vi "SQLDisconnect.vi"(4 "error in (no error)":errorcluster, 7 "InputHandle":i32) -> (0 "error out":errorcluster, 3 "OutputHandle":i32)   [LabVIEW 2011]
doc: "Se déconnecte de la base de donnée référencée par le lien"
uses:
  Odbc32.dll
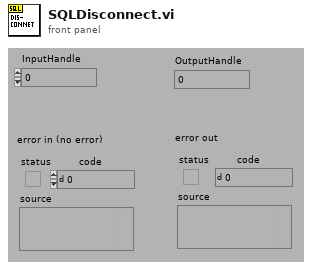
[diagram p1: front panel]
types:
  T1 = enum16{"NOPE", "SQL_HANDLE_ENV", "SQL_HANDLE_DBC", "SQL_HANDLE_STMT", "SQL_HANDLE_DESC"}
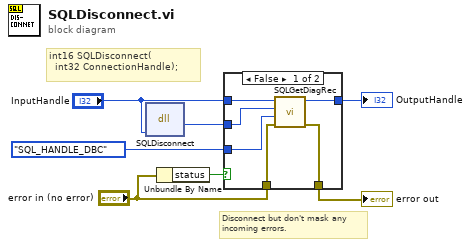
[diagram p0: block diagram]
diagram:
  # "Disconnect but don't mask any\nincoming errors."
  # "int16 SQLDisconnect(\n  int32 ConnectionHandle);"
  n1 = dll-call lib="Odbc32.dll" fn="SQLDisconnect"("ConnectionHandle"="InputHandle") -> (w4:i16)  [unwired: 4 in, 2 out]
  n2 = Unbundle By Name("error in (no error)") -> ("status"=w2:bool)
  n3 = case shown="False" w2 {
    tunnel: "error in (no error)" -> [w13 w15]
    tunnel: [w12 w15] -> w7
    tunnel: "InputHandle" -> [w11 w14]
    tunnel: [w10 w14] -> w5
    tunnel: w4 -> [w9 _]
    tunnel: T1."SQL_HANDLE_DBC" ("HandleType") -> [w8 _]
    frame False {
      n4 = call "SQLGetDiagRec.vi"("error in (no error)"=w13, "HandleType"=w8, "Status (SQL_SUCCESS=0)"=w9, "Input Handle"=w11) -> ("error out"=w12:errorcluster, "Output Handle"=w10:i32)  [unwired: 2 out]
    }
    frame True {
    }
  }
  "OutputHandle" <- w5
  "error out" <- w7
